vi "CreateWaveformArray.vi"(11 "bufferSize":dbl) -> (3 "initialized array":waveform(dbl)[](array[waveform]))   [LabVIEW 2016]
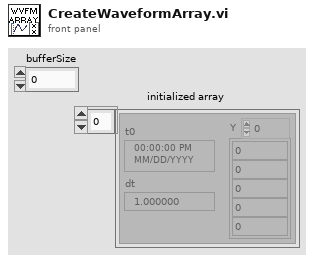
[diagram p1: front panel]
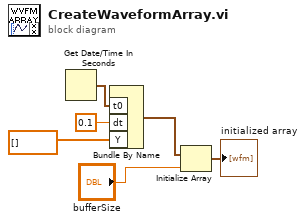
[diagram p0: block diagram]
diagram:
  n1 = Get Date/Time In Seconds() -> (seconds since 1Jan1904=w3:timestamp)
  n2 = Bundle By Name("t0"=w3, "dt"=0.1, "Y"=dbl[] []) -> (w6:waveform(dbl))  [unwired: 1 in]
  n3 = Initialize Array(w6, "bufferSize") -> (→"initialized array":waveform(dbl)[])
